vi "TestPFGVReadUIDs.vi"() -> (0 "error out":errorcluster, 2 "Pass":bool)   [LabVIEW 2015]
uses:
  TypeDef/RoomsActionEnum.ctl
  TypeDef/PersonnelActions.ctl
  LVClasses/Flags/Flags.lvclass
  LVClasses/Room/Room.lvclass
panel:
  out "PUIDs Init":string
  out "PUIDs Personnel":string
  in  "PUID":string="d1"
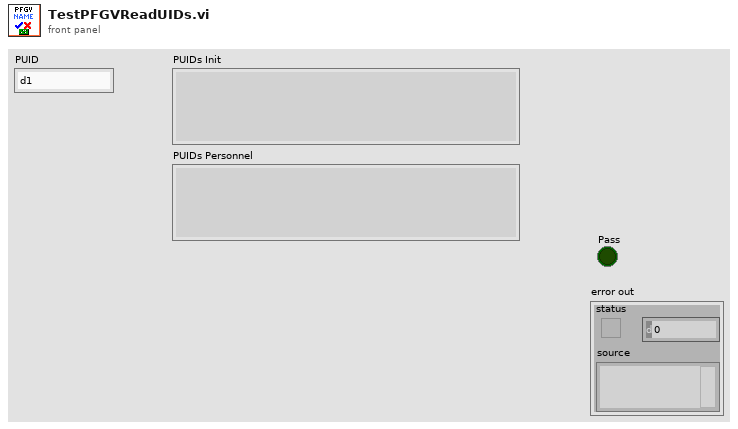
[diagram p1: front panel]
types:
  T1 = typedef "PersonnelActions.ctl" = enum16{"Init", "Read Personnel", "Add Personnel", "Remove Personnel", "Read Name", "Write Name", "Read Role", "Write Role", "Read Requests", "Add Requests", "Remove Requests", "Read PUIDs"}
  T2 = typedef "RoomsActionEnum.ctl" = enum16{"Init", "Add Room", "Remove Room", "Read Room", "Read Flag", "Read Flag State", "Write Flag State", "Read Flag Color", "Write Flag Color", "Read Bed Vacant", "Write Bed Vacant", "Read Personnel", "Add Personnel", "Remove Personnel", "Read Requests", "Add Request", "Remove Request", "Read Beacon ID", "Write Beacon ID", "Write Bed URL", "Read Bed URL", "Read Rooms Numbers", "Write Flag"}
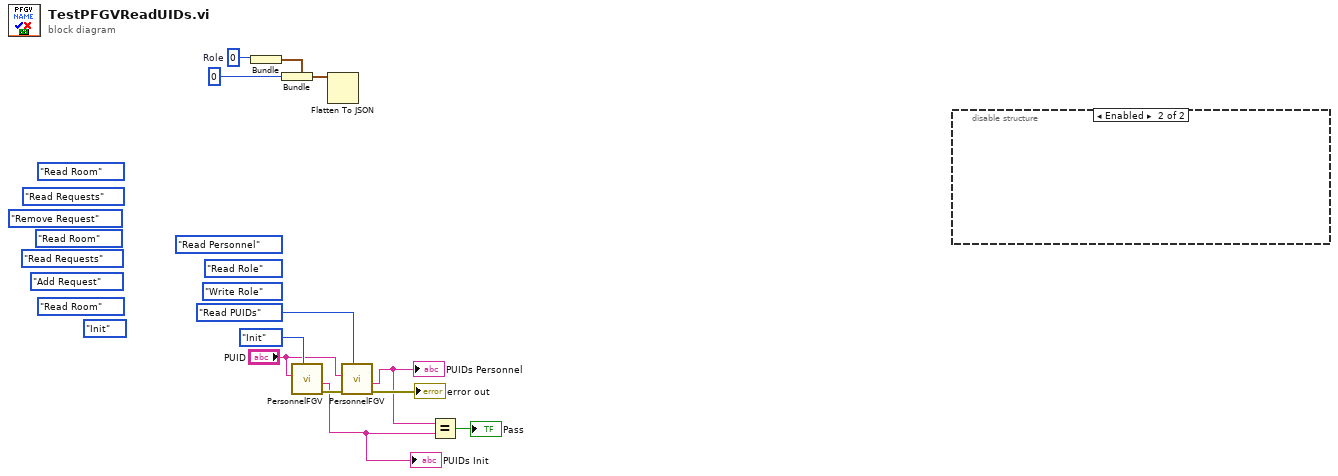
[diagram p0: block diagram]
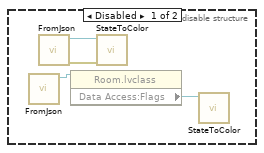
[diagram p2: hidden frame]
diagram:
  (unwired) PersonnelActions."Read Personnel" ("Actions")
  (unwired) PersonnelActions."Read Role" ("Actions")
  (unwired) PersonnelActions."Write Role" ("Actions")
  (unwired) RoomsActionEnum."Read Requests"
  (unwired) RoomsActionEnum."Remove Request"
  w11 = 0  # Role
  (unwired) RoomsActionEnum."Add Request"
  (unwired) RoomsActionEnum."Read Room"
  (unwired) RoomsActionEnum."Read Requests" ("Actions")
  (unwired) RoomsActionEnum."Read Room"
  (unwired) RoomsActionEnum."Read Room"
  (unwired) RoomsActionEnum."Init"
  n1 = Bundle("Role"=w11) -> (w10:cluster{"Role":i32})  [unwired: 1 in]
  n2 = Bundle(cluster=w10, "Role"=0 ("Request")) -> (w9:cluster{"Role":i32})
  n3 = call "PersonnelFGV.vi"("Actions"=PersonnelActions."Init", "PUID"="PUID") -> ("error out"=w12:errorcluster, "Data Out"=w2:string)  [unwired: 8 in]
  "PUIDs Init" <- w2
  n4 = Flatten To JSON(anything=w9) -> ()  [unwired: 2 in, 2 out]
  n5 = call "PersonnelFGV.vi"("Actions"=PersonnelActions."Read PUIDs", "error in (no error)"=w12, "PUID"="PUID") -> ("error out"=→"error out":errorcluster, "Data Out"=w3:string)  [unwired: 7 in]
  "PUIDs Personnel" <- w3
  n6 = Equal?(x=w3, y=w2) -> (x = y?=→"Pass":bool)
  n7 = disable-structure shown="Enabled" {
    frame Disabled {
      n8 = call "FromJson.vi"() -> ("Room out"=w14:refnum<class "Room.lvclass">)  [unwired: 10 in, 1 out]
      n9 = call "FromJson.vi"() -> ("error out"=w16:errorcluster, "Flags out"=w15:refnum<class "Flags.lvclass">)  [unwired: 10 in]
      n10 = property class="Room.lvclass"(reference=w14) -> ("Data Access:Flags"=w13:refnum<class "Flags.lvclass">)  [unwired: 1 in, 2 out]
      n11 = call "StateToColor.vi"("error in (no error)"=w16, "Flags in"=w15) -> ()  [unwired: 7 in, 3 out]
      n12 = call "StateToColor.vi"("Flags in"=w13) -> ()  [unwired: 8 in, 3 out]
    }
    frame Enabled {
    }
  }
